vi "PicoScope2000aUnitInfo.vi"(0 "error in (no error)":errorcluster, 1 "handle in":i16, 2 "Mode":u16(ring) items=["Dialog On Error", "no dialog - CloseUnit and Stop", "no dialog - Continue", "no dialog - Stop"]) -> (3 "error out":errorcluster, 4 "PICO_STATUS":u32, 5 "handle out":i16, 6 "Unit Info":T1)   [LabVIEW 2010]
uses:
  ps2000a.dll
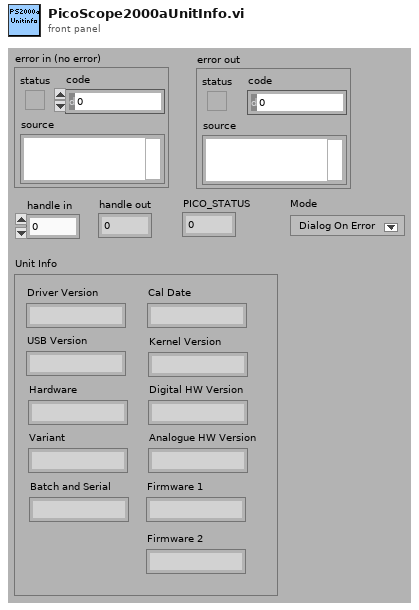
[diagram p1: front panel]
types:
  T1 = cluster{"Driver Version":string, "USB Version":string, "Hardware":string, "Variant":string, "Batch and Serial":string, "Cal Date":string, "Kernel Version":string, "Digital HW Version":string, "Analogue HW Version":string, "Firmware 1":string, "Firmware 2":string}
  T2 = cluster{"status":bool, "code":u32, "source":string}
  T3 = cluster{"[0]":string, "[1]":string, "[2]":string, "[3]":string, "[4]":string, "[5]":string, "[6]":string, "[7]":string, "[8]":string, "[9]":string, "[10]":string}
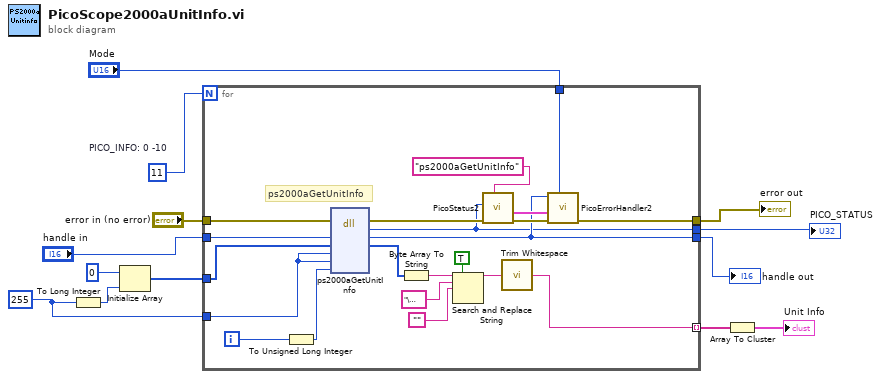
[diagram p0: block diagram]
diagram:
  w3 = i16 255 ("dimension size")
  w12 = 11  # PICO_INFO: 0 -10
  n1 = To Long Integer(number=w3) -> (32bit integer=w2:i32)
  n2 = Initialize Array(u8 0 ("U8"), w2) -> (w4:u8[])
  n3 = for {
    N: w12 -> [_]
    tunnel: "handle in" -> [w34]
    tunnel: [w25] -> w8 mode=indexing
    tunnel: "error in (no error)" -> [w32]
    tunnel: [w17] -> w10
    tunnel: [w16] -> w6
    tunnel: [w15] -> w9
    tunnel: w4 -> [w23]
    tunnel: w3 -> [w22]
    tunnel: "Mode" -> [w14]
    i -> [w33]
    # "ps2000aGetUnitInfo"
    n4 = To Unsigned Long Integer(number=w33) -> (unsigned 32bit integer=w31:u32)
    n5 = dll-call lib="PS2000a.dll" fn="ps2000aGetUnitInfo"(error in=w32, "handle"=w34, "unitInfo"=w23, "stringLength"=w22, "requiredSize"=w22, "PICO_INFO"=w31) -> (error out=w18:errorcluster, "PICO_STATUS"=w15:u32, "handle"=w17:i16, "unitInfo"=w24:u8[])  [unwired: 5 in, 1 out]
    n6 = Byte Array To String(unsigned byte array=w24) -> (string=w29:string)
    n7 = Search and Replace String(replace all?=TRUE ("replace all? (F)"), input string=w29, search string="\u0000", replace string="") -> (result string=w28:string)  [unwired: 4 in, 3 out]
    n8 = call "PicoStatus2.vi"("PICO source"="ps2000aGetUnitInfo" ("source"), "Error in"=w18, "PICO STATUS"=w15) -> ("error out"=w21:errorcluster, "PICO_STATUS out"=w19:T2)  [unwired: 5 in]
    n9 = call <vilib>:"Trim Whitespace.vi"("string"=w28) -> ("trimmed string"=w25:string)  [unwired: 1 in]
    n10 = call "PicoErrorHandler2.vi"("Mode"=w14, "error in (no error)"=w21, "PICO_STATUS in"=w19, "handle In"=w17) -> ("error out"=w16:errorcluster)  [unwired: 7 in]
  }
  "error out" <- w6
  "handle out" <- w10
  "PICO_STATUS" <- w9
  n11 = Array To Cluster(array=w8) -> (cluster=→"Unit Info":T3)
